vi "ReadingData_Module.vi"() -> ()   [LabVIEW 2020]
uses:
  State2.ctl
  V&T_Data.ctl
  D&P_Data.ctl
  <vilib>/Instr/_visa.llb/VISA Configure Serial Port (Instr).vi
  <vilib>/Utility/file.llb/Write Delimited Spreadsheet (DBL).vi
panel:
  out "Sensor Locked?":bool
  out "Q OutOfRange?":bool
  out "Density and Pressure Graph":T1(graph)
  out "Viscosity and Temperature Graph":T1(graph)
  out "StateR":T2=enum."ReadSerial"
  in  "Save Button":bool
  in  "Rec Button":bool
  in  "VISA resource name (COM)":refnum<visa-resource-name>="CNCB0"
  in  "stop":bool
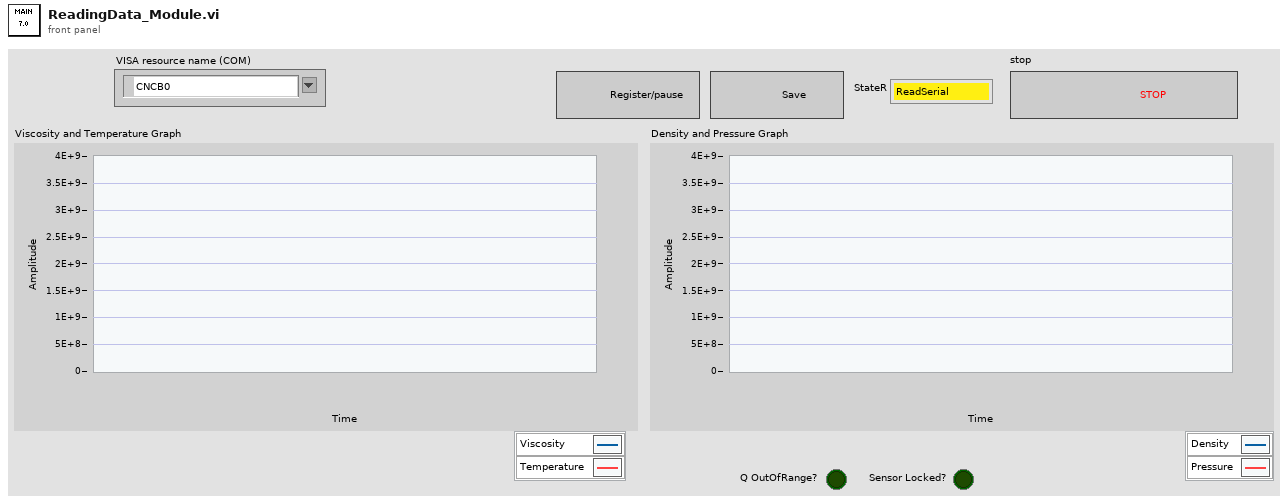
[diagram p1: front panel]
types:
  T1 = cluster{"seconds since 1Jan1904":timestamp, dbl, dbl}[]
  T2 = typedef "State2.ctl" = enum16{"Initialize", "ReadSerial", "ShowData", "SaveData", "Finalize"}
  T3 = typedef "D&P_Data.ctl" = cluster{"time":timestamp, "Density":dbl, "Pressure":dbl}
  T4 = typedef "V&T_Data.ctl" = cluster{"time":timestamp, "Viscosity":dbl, "Temperature":dbl}
  T5 = enum8{"Enabled", "Disabled", "Disabled and Grayed Out"}
  T6 = enum16{"open", "replace", "create", "open or create", "replace or create", "replace or create with confirmation"}
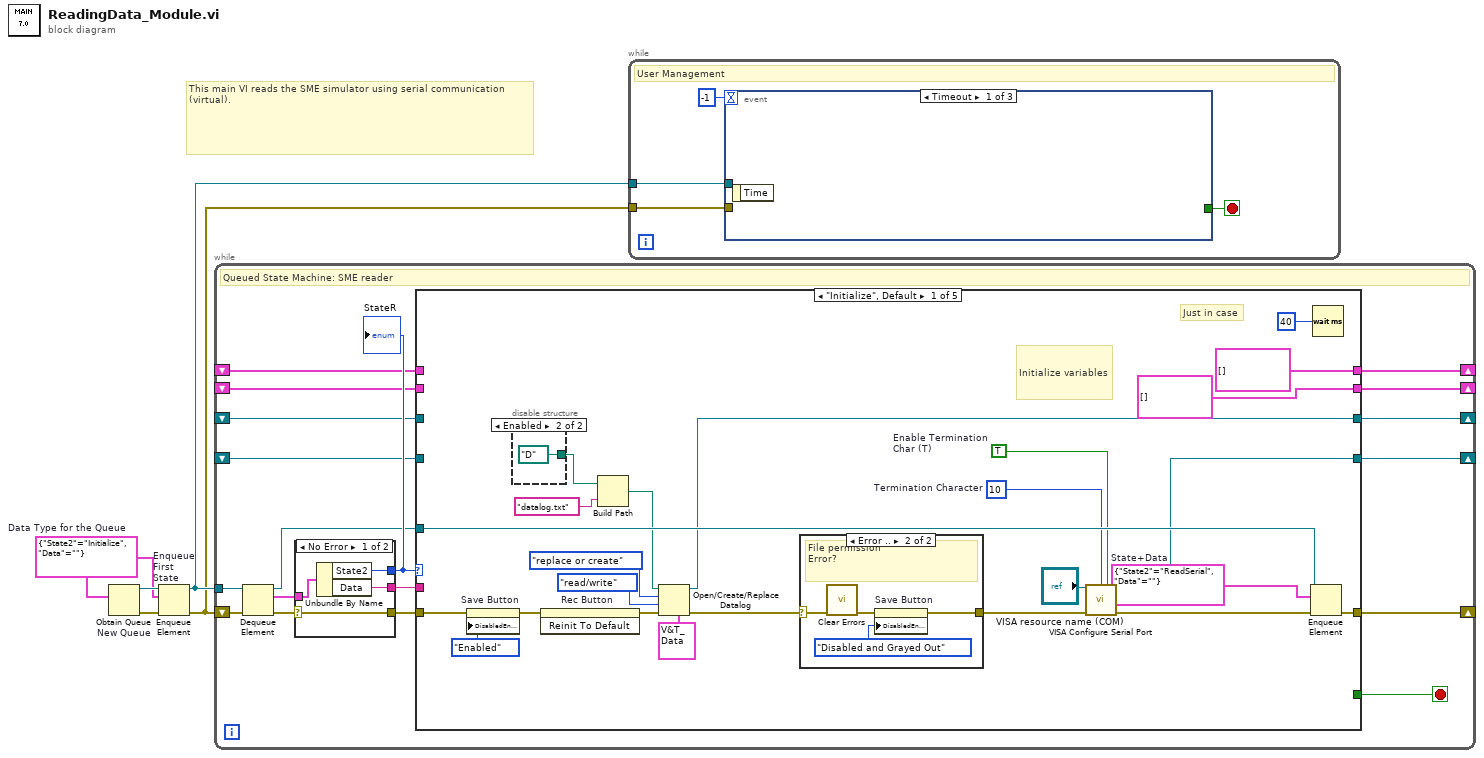
[diagram p0: block diagram]
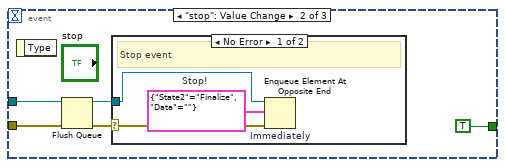
[diagram p2: hidden frame]
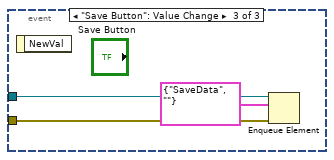
[diagram p4: hidden frame]
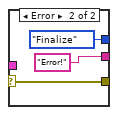
[diagram p5: hidden frame]
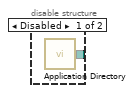
[diagram p6: hidden frame]
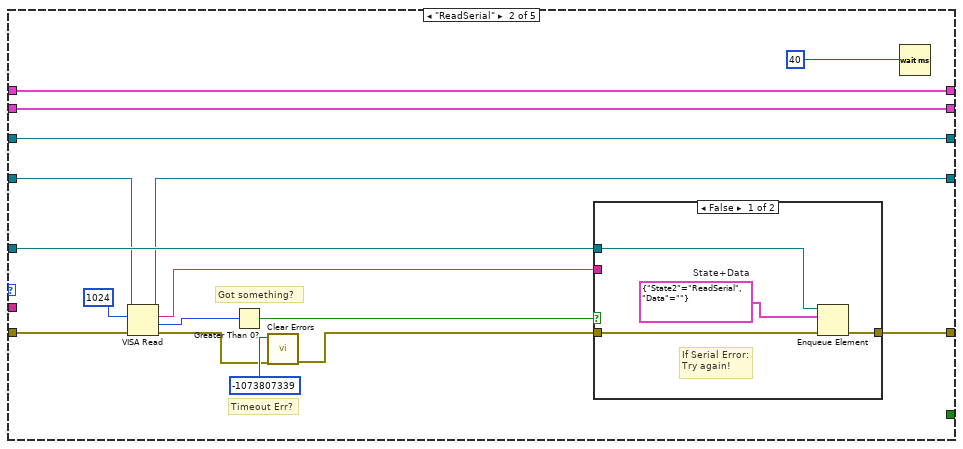
[diagram p8: hidden frame]
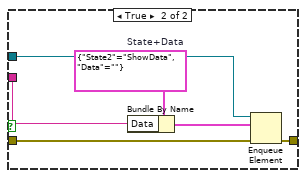
[diagram p9: hidden frame]
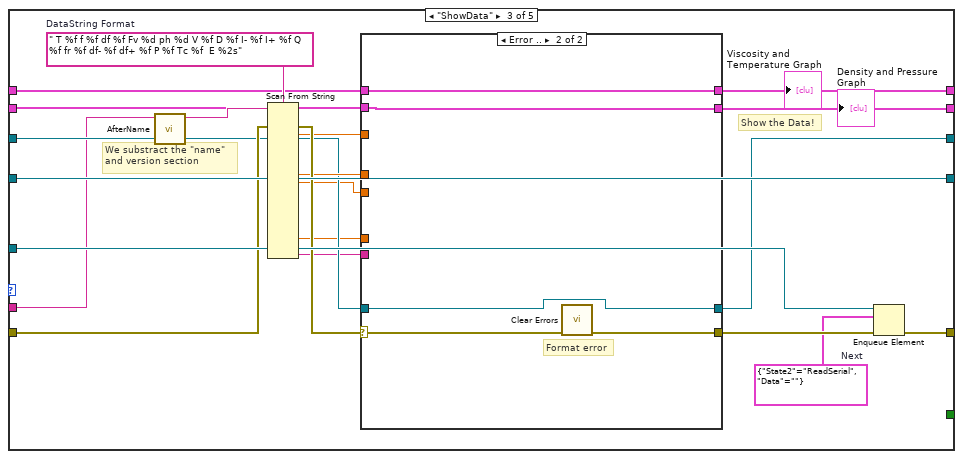
[diagram p10: hidden frame]
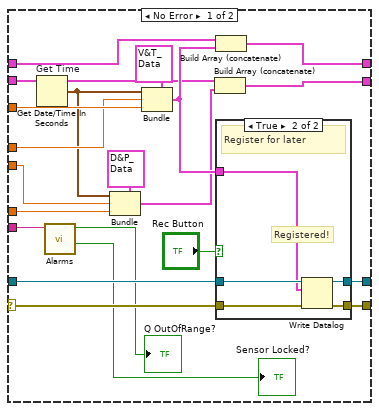
[diagram p11: hidden frame]
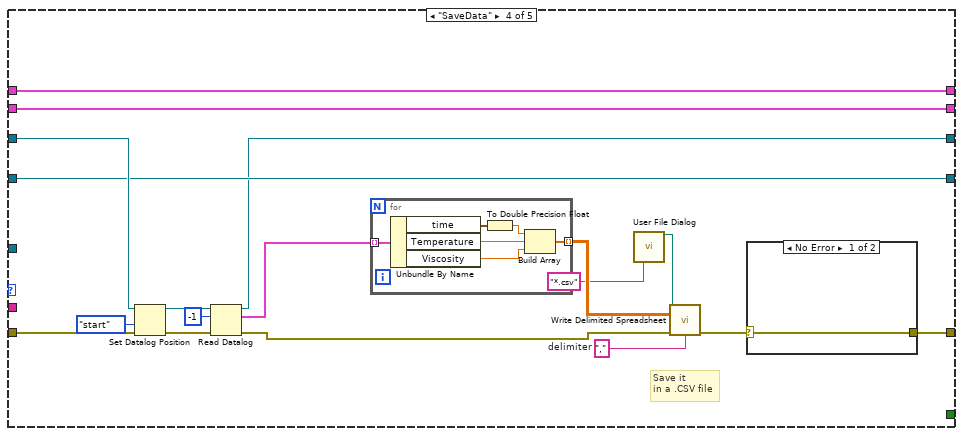
[diagram p13: hidden frame]
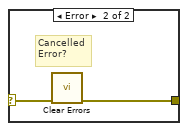
[diagram p14: hidden frame]
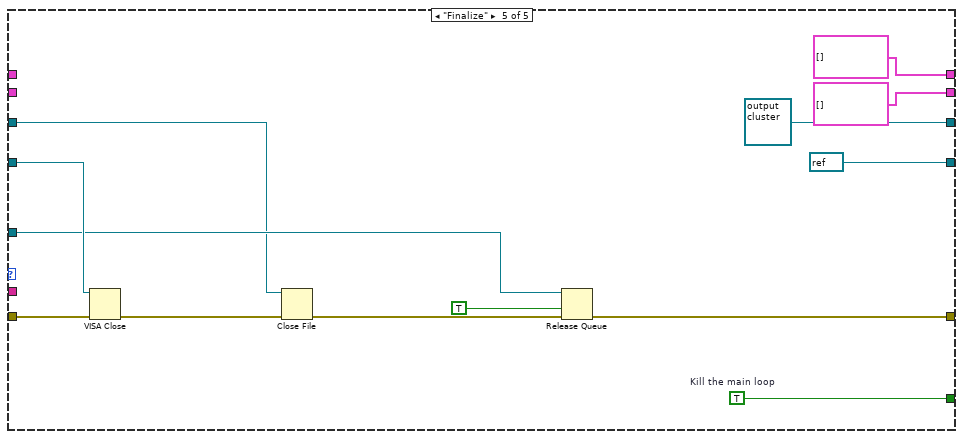
[diagram p15: hidden frame]
diagram:
  w4 = cluster{"State2":T2, "Data":string} {"State2"=enum."Initialize", "Data"=""}  # Data Type for the Queue
  # "This main VI reads the SME simulator using serial communication (virtual)."
  n1 = Obtain Queue "New Queue"(element data type=w4) -> (queue out=w5:refnum<queue>, error out=w3:errorcluster)  [unwired: 4 in, 1 out]
  n2 = Enqueue Element "Enqueue\nFirst\nState"(queue=w5, element=w4, error in (no error)=w3) -> (queue out=w2:refnum<queue>, error out=w1:errorcluster)  [unwired: 1 in, 1 out]
  n3 = while {
    shift-right: [w20] -> _
    shift-left: w1 -> [w16]
    shift-right: [w19] -> _
    shift-left: _ -> [w18]
    tunnel: w2 -> [w17]
    shift-right: [w10] -> _
    shift-left: _ -> [w11]
    shift-right: [w9] -> _
    shift-left: _ -> [w8]
    shift-right: [w6] -> _
    shift-left: _ -> [w7]
    stop <- w13 stop-if-true
    # "Queued State Machine: SME reader"
    n4 = Dequeue Element(queue=w17, error in (no error)=w16) -> (queue out=w12:refnum<queue>, element=w14:cluster{"State2":T2, "Data":string}, error out=w15:errorcluster)  [unwired: 1 in, 1 out]
    n5 = case shown="No Error" w15 {
      selector: w15 -> [w24 w29]
      tunnel: w14 -> [w27 _]
      tunnel: [w26 State2."Finalize" ("State2")] -> w23
      tunnel: [w25 "Error!" ("Data")] -> w22
      tunnel: [w24 w29] -> w21
      frame No Error {
        n6 = Unbundle By Name(w27) -> ("State2"=w26:T2, "Data"=w25:string)
      }
      frame Error {
      }
    }
    "StateR" <- w23
    n7 = case shown="\"Initialize\", Default" w23 {
      tunnel: w22 -> [_ _ w91 _ _]
      tunnel: w21 -> [w35 w70 w103 w158 w180]
      tunnel: [w53 w76 w106 w148 w177] -> w20
      tunnel: [w49 w68 w108 w145 refnum<visa-resource-name> refnum ("VISA resource name")] -> w19
      tunnel: w18 -> [_ w71 w108 w145 w181]
      tunnel: [_ _ _ _ w178] -> w13
      tunnel: w12 -> [w54 w77 w107 _ w176]
      tunnel: w11 -> [_ w75 w99 w159 _]
      tunnel: [T4[] [] w75 w95 w159 T4[] []] -> w10
      tunnel: [w42 w63 w96 w144 refnum<k1> refnum] -> w9
      tunnel: w8 -> [_ w63 w97 w147 w173]
      tunnel: w7 -> [_ w62 w89 w142 _]
      tunnel: [T3[] [] w62 w88 w142 T3[] []] -> w6
      frame "Initialize", Default {
        w47 = cluster{"State2":T2, "Data":string} {"State2"=enum."ReadSerial", "Data"=""}  # State+Data
        w51 = u8 10  # Termination Character
        w52 = TRUE  # Enable Termination Char (T)
        # "Just in case"
        # "Initialize variables"
        n8 = property on="Save Button" class="Bool"(error in=w35, "DisabledEnum"=T5."Enabled" ("Disabled")) -> (error out=w34:errorcluster)  [unwired: 1 in, 1 out]
        n9 = disable-structure shown="Enabled" {
          disable-tunnel: [w55 path "D:/" ("Application Directory")] -> w45
          frame Disabled {
            n10 = call <vilib>:"Application Directory.vi"() -> ("Application Directory"=w55:path)
          }
          frame Enabled {
          }
        }
        n11 = invoke on="Rec Button" class="Bool (strict)" method="Reinit To Default"(error in=w34) -> (error out=w33:errorcluster)  [unwired: 2 in, 2 out]
        n12 = Build Path(base path=w45, name or relative path="datalog.txt") -> (appended path=w43:path)
        n13 = Open/Create/Replace Datalog(5:T4 {"time"=timestamp(0 s since 1904-01-01), "Viscosity"=0.0, "Temperature"=0.0} ("output cluster"), 8:w33, 9:enum16{"read/write", "read-only", "write-only"}."read/write" ("access (0:read/write)"), 10:T6."replace or create" ("operation (0:open)"), 11:w43) -> (0:w40:errorcluster, 3:w42:refnum<k1>)  [unwired: 1 in, 1 out]
        n14 = case shown="Error .." w40 {
          selector: w40 -> [w57 w61]
          tunnel: [w57 w59] -> w39
          frame No Error {
          }
          frame Error {
            # "File permission\nError?"
            n15 = call <vilib>:"Clear Errors.vi"("error in (no error)"=w61) -> ("error out"=w60:errorcluster)  [unwired: 5 in, 1 out]
            n16 = property on="Save Button" class="Bool"(error in=w60, "DisabledEnum"=T5."Disabled and Grayed Out" ("Disabled")) -> (error out=w59:errorcluster)  [unwired: 1 in, 1 out]
          }
        }
        n17 = call-poly "VISA Configure Serial Port"("VISA resource name"="VISA resource name (COM)", "termination char\n(0xA = '\\n' = LF)"=w51, "Enable Termination\nChar (T)"=w52, "error in (no error)"=w39) -> ("VISA resource name out"=w49:refnum<visa-resource-name>, "error out"=w48:errorcluster)  [unwired: 10 in]
        n18 = Enqueue Element(queue=w54, element=w47, error in (no error)=w48) -> (error out=w53:errorcluster)  [unwired: 1 in, 2 out]
        n19 = Wait (ms)(milliseconds to wait=u32 40) -> ()  [unwired: 1 out]
      }
      frame "ReadSerial" {
        # "Timeout Err?"
        # "Got something?"
        n20 = VISA Read(VISA resource name=w71, byte count=u32 1024, error in (no error)=w70) -> (VISA resource name out=w68:refnum<visa-resource-name>, read buffer=w67:string, return count=w72:u32, error out=w65:errorcluster)
        n21 = Greater Than 0?(x=w72) -> (x > 0?=w69:bool)
        n22 = call <vilib>:"Clear Errors.vi"("error in (no error)"=w65, "specific error code to clear (0: all)"=-1073807339 ("y")) -> ("error out"=w64:errorcluster)  [unwired: 4 in, 1 out]
        n23 = case shown="False" w69 {
          tunnel: w77 -> [w81 w87]
          tunnel: [w80 w86] -> w76
          tunnel: w64 -> [w78 w85]
          tunnel: w67 -> [_ w83]
          frame False {
            w79 = cluster{"State2":T2, "Data":string} {"State2"=enum."ReadSerial", "Data"=""}  # State+Data
            # "If Serial Error:\nTry again!"
            n24 = Enqueue Element(queue=w81, element=w79, error in (no error)=w78) -> (error out=w80:errorcluster)  [unwired: 1 in, 2 out]
          }
          frame True {
            w84 = cluster{"State2":T2, "Data":string} {"State2"=enum."ShowData", "Data"=""}  # State+Data
            n25 = Bundle By Name(cluster=w84, "Data"=w83) -> (w82:cluster{"State2":T2, "Data":string})
            n26 = Enqueue Element(queue=w87, element=w82, error in (no error)=w85) -> (error out=w86:errorcluster)  [unwired: 1 in, 2 out]
          }
        }
        n27 = Wait (ms)(milliseconds to wait=u32 40) -> ()  [unwired: 1 out]
      }
      frame "ShowData" {
        w101 = cluster{"State2":T2, "Data":string} {"State2"=enum."ReadSerial", "Data"=""}  # Next
        w104 = " T %f f %f df %f Fv %d ph %d V %f D %f I- %f I+ %f Q %f fr %f df- %f df+ %f P %f Tc %f  E %2s"  # DataString Format
        # "We substract the \"name\"\nand version section"
        # "Show the Data!"
        n28 = call "AfterName.vi"("The String"=w91) -> ("after \"Name\""=w90:string)  [unwired: 10 in]
        n29 = Scan From String(format string=w104, input string=w90, error in=w103) -> (error out=w102:errorcluster, output 1=w100:dbl, output 6=w98:dbl, output 7=w94:dbl, output 14=w93:dbl, output 16=w92:string)  [unwired: 28 in, 2 out]
        n30 = case shown="Error .." w102 {
          selector: w102 -> [w127 w141]
          tunnel: [w124 w140] -> w105
          tunnel: w99 -> [w128 w139]
          tunnel: w100 -> [w120 _]
          tunnel: [w129 w139] -> w95
          tunnel: w98 -> [w119 _]
          tunnel: w97 -> [w126 w138]
          tunnel: [w125 w138] -> w96
          tunnel: w94 -> [w110 _]
          tunnel: w93 -> [w109 _]
          tunnel: w92 -> [w113 _]
          tunnel: w89 -> [w116 w137]
          tunnel: [w114 w137] -> w88
          frame No Error {
            n31 = Get Date/Time In Seconds "Get Time"() -> (seconds since 1Jan1904=w117:timestamp)
            n32 = call "Alarms.vi"("Error"=w113) -> ("SensorLocked?"=→"Sensor Locked?":bool, "Q_OutOfRange?"=→"Q OutOfRange?":bool)  [unwired: 9 in]
            n33 = Bundle(cluster=T3 {"time"=timestamp(0 s since 1904-01-01), "Density"=0.0, "Pressure"=0.0} ("D&P Data"), "time"=w117, "Density"=w110, "Pressure"=w109) -> (w115:T3)
            n34 = Bundle(cluster=T4 {"time"=timestamp(0 s since 1904-01-01), "Viscosity"=0.0, "Temperature"=0.0} ("output cluster"), "time"=w117, "Viscosity"=w119, "Temperature"=w120) -> (w121:T4)
            n35 = Build Array (concatenate)(w116, w115) -> (w114:T3[])
            n36 = Build Array (concatenate)(w128, w121) -> (w129:T4[])
            n37 = case shown="True" "Rec Button" {
              tunnel: w127 -> [w130 w136]
              tunnel: w126 -> [w131 w135]
              tunnel: [w131 w134] -> w125
              tunnel: [w130 w133] -> w124
              tunnel: w121 -> [_ w132]
              frame False {
                # "Pause or \nhasn't started"
              }
              frame True {
                # "Registered!"
                # "Register for later"
                n38 = Write Datalog(4:w136, 6:w132, 7:w135) -> (0:w133:errorcluster, 3:w134:refnum<k1>)
              }
            }
          }
          frame Error {
            # "Format error"
            n39 = call <vilib>:"Clear Errors.vi"("error in (no error)"=w141) -> ("error out"=w140:errorcluster)  [unwired: 5 in, 1 out]
          }
        }
        "Viscosity and Temperature Graph" <- w95
        "Density and Pressure Graph" <- w88
        n40 = Enqueue Element(queue=w107, element=w101, error in (no error)=w105) -> (error out=w106:errorcluster)  [unwired: 1 in, 2 out]
      }
      frame "SaveData" {
        w143 = ","  # delimiter
        # "Save it\nin a .CSV file"
        n41 = Set Datalog Position(4:w158, 5:enum16{"start", "end", "current"}."start" ("from (0:start)"), 7:w147) -> (0:w155:errorcluster, 3:w156:refnum<k1>)  [unwired: 1 in]
        n42 = Read Datalog(4:w155, 6:-1 ("count (1)"), 7:w156) -> (0:w150:errorcluster, 2:w154:T4[], 3:w144:refnum<k1>)
        n43 = for {
          tunnel: w154 -> [w168] mode=indexing
          tunnel: [w163] -> w153 mode=indexing
          n44 = Unbundle By Name(w168) -> ("time"=w165:timestamp, "Temperature"=w166:dbl, "Viscosity"=w167:dbl)
          n45 = To Double Precision Float(number=w165) -> (double precision float=w164:dbl)
          n46 = Build Array(w164, w166, w167) -> (w163:dbl[])
        }
        n47 = call "User File Dialog"("pattern (all files)"="*.csv") -> ("selected path"=w151:path)  [unwired: 11 in, 3 out]
        n48 = call-poly <vilib>:"Write Delimited Spreadsheet.vi"("file path (dialog if empty)"=w151, "2D data"=w153, "error in (no error)"=w150, "delimiter (\\t)"=w143) -> ("error out"=w149:errorcluster)  [unwired: 10 in, 1 out]
        n49 = case shown="No Error" w149 {
          selector: w149 -> [w160 w162]
          tunnel: [w160 w161] -> w148
          frame No Error {
          }
          frame Error {
            # "Cancelled\nError?"
            n50 = call <vilib>:"Clear Errors.vi"("error in (no error)"=w162) -> ("error out"=w161:errorcluster)  [unwired: 5 in, 1 out]
          }
        }
      }
      frame "Finalize" {
        w178 = TRUE  # Kill the main loop
        n51 = VISA Close(VISA resource name=w181, error in (no error)=w180) -> (error out=w172:errorcluster)
        n52 = Close File(refnum=w173, error in=w172) -> (error out=w171:errorcluster)  [unwired: 1 out]
        n53 = Release Queue(queue=w176, force destroy? (F)=TRUE, error in (no error)=w171) -> (error out=w177:errorcluster)  [unwired: 2 out]
      }
    }
  }
  n54 = while {
    tunnel: w2 -> [w183]
    tunnel: w1 -> [w182]
    stop <- w184 stop-if-true
    # "User Management"
    n55 = event shown="[0] Timeout" {
      selector: _ -> [_ _ _]
      dyn-events: _ -> [_ _ _]
      timeout: -1 -> [_ _ _]
      tunnel: [_ TRUE _] -> w184
      tunnel: w183 -> [_ w188 w196]
      tunnel: w182 -> [_ w189 w194]
      event Timeout {
        n56 = event-data() -> ()  [unwired: 1 in, 1 out]
      }
      event "stop": Value Change {
        n57 = event-data() -> ()  [unwired: 1 in, 1 out]
        n58 = Flush Queue(queue=w188, error in (no error)=w189) -> (queue out=w187:refnum<queue>, error out=w186:errorcluster)  [unwired: 1 out]
        n59 = case shown="No Error" w186 {
          selector: w186 -> [w192 _]
          tunnel: w187 -> [w193 _]
          frame No Error {
            w191 = cluster{"State2":T2, "Data":string} {"State2"=enum."Finalize", "Data"=""}  # Stop!
            # "Stop event"
            n60 = Enqueue Element At Opposite End "Immediately"(queue=w193, element=w191, error in (no error)=w192) -> ()  [unwired: 1 in, 3 out]
          }
          frame Error {
            # "Already dead"
          }
        }
      }
      event "Save Button": Value Change {
        n61 = event-data() -> ()  [unwired: 1 in, 1 out]
        n62 = Enqueue Element(queue=w196, element=cluster{"State2":T2, "Data":string} {"State2"=enum."SaveData", "Data"=""}, error in (no error)=w194) -> ()  [unwired: 1 in, 3 out]
      }
    }
  }
